vi "Overwrite Item.vi"(8 "error in (no error)":errorcluster, 9 "BetterTreeItem in":refnum<class "BetterItem.lvclass">, 10 "TreeItem Index":i32, 11 "BetterTreeHandle in":refnum<class "BetterTreeHandle.lvclass">) -> (0 "error out":errorcluster, 3 "BetterTreeHandle out":refnum<class "BetterTreeHandle.lvclass">)   [LabVIEW 2020, in "BetterDragAndDrop.lvlib" / "BetterTreeHandle.lvclass"]
uses:
  BetterTreeHandle.lvclass
  C:/DSCE code/Open-source/betterdraganddrop_GIT/Source/Classes/BetterHandle/BetterHandle.lvclass
  BetterTreeItem/BetterItem.lvclass
  BetterHandle/BetterHandle.lvclass/BetterHandle.ctl
  BetterTreeHandle.lvclass/BetterTreeHandle.ctl
  BetterTreeItem/BetterItem.lvclass/BetterItem.ctl
  BetterHandle/BetterHandle.lvclass
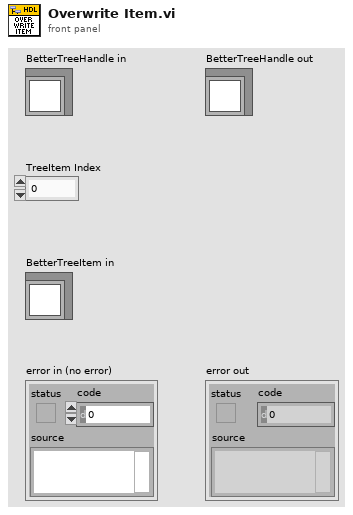
[diagram p1: front panel]
types:
  T1 = typedef "BetterDragAndDrop.lvlib/BetterTreeHandle.lvclass/TreeItem.ctl" = cluster{"Left Cell String":string, "Child Text":string[], "Child Tag":string, "Item Indent":i32, "Child Only?":bool, "Glyph Index":i32, "Font Color":u32}
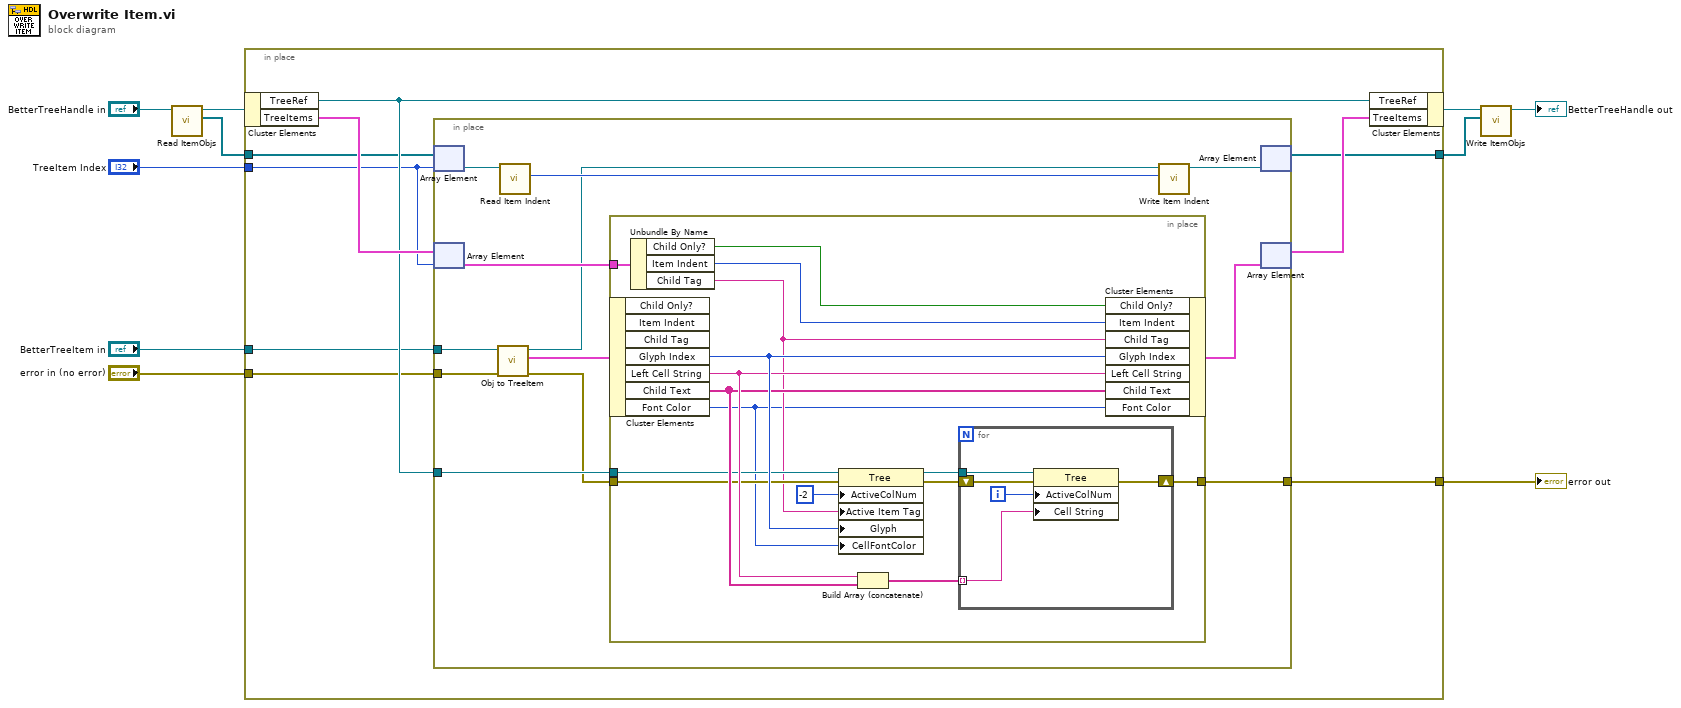
[diagram p0: block diagram]
diagram:
  n1 = call "Read ItemObjs.vi"("BetterHandle in"="BetterTreeHandle in") -> ("ItemObjs"=w4:refnum<class "BetterItem.lvclass">[], "BetterHandle out"=w5:refnum<class "BetterTreeHandle.lvclass">)  [unwired: 9 in]
  n2 = in-place {
    in-place-border: "error in (no error)" -> [w16]
    in-place-border: [w15] -> w8
    in-place-border: "TreeItem Index" -> [w14]
    in-place-border: "BetterTreeItem in" -> [w13]
    in-place-border: w4 -> [w12]
    in-place-border: [w11] -> w1
    n3 = in-place-cluster #1(w5) -> ("TreeRef"=w17:refnum<vi>, "TreeItems"=w19:T1[])
    n4 = in-place {
      in-place-border: w17 -> [w31]
      in-place-border: w13 -> [w24]
      in-place-border: w16 -> [w21]
      in-place-border: [w30] -> w15
      n5 = in-place-array #2(w12, w14) -> (w27:refnum<class "BetterItem.lvclass">)
      n6 = in-place-array #3(w19, w14) -> (w29:T1)
      n7 = call "Obj to TreeItem.vi"("error in (no error)"=w21, "BetterTreeItem in"=w24) -> ("error out"=w20:errorcluster, "Tree Control Item"=w22:T1, "BetterTreeItem out"=w23:refnum<class "BetterItem.lvclass">)  [unwired: 7 in]
      n8 = call "Read Item Indent.vi"("BetterTreeItem in"=w27) -> ("Item Indent"=w25:i32)  [unwired: 9 in, 1 out]
      n9 = in-place {
        in-place-border: w31 -> [w36]
        in-place-border: w20 -> [w35]
        in-place-border: [w43] -> w30
        in-place-border: w29 -> [w42]
        n10 = in-place-cluster #4(w22) -> ("Glyph Index"=w41:i32, "Left Cell String"=w40:string, "Child Text"=w39:string[], "Font Color"=w32:u32)  [unwired: 3 out]
        n11 = Unbundle By Name(w42) -> ("Child Only?"=w38:bool, "Item Indent"=w37:i32, "Child Tag"=w34:string)
        n12 = property class="Tree"(reference=w36, error in=w35, "ActiveColNum"=-2 ("Active Cell:Active Column Number"), "Active Item Tag"=w34, "Glyph"=w41, "CellFontColor"=w32) -> (reference out=w46:refnum<vi>, error out=w44:errorcluster)
        n13 = Build Array (concatenate)(w40, w39) -> (w45:string[])
        n14 = for {
          tunnel: w46 -> [w51]
          tunnel: w45 -> [w49] mode=indexing
          shift-right: [w47] -> w43
          shift-left: w44 -> [w48]
          i -> [w50]
          n15 = property class="Tree"(reference=w51, error in=w48, "ActiveColNum"=w50, "Cell String"=w49) -> (error out=w47:errorcluster)  [unwired: 1 out]
        }
        n16 = in-place-cluster #4("Child Only?"=w38, "Item Indent"=w37, "Child Tag"=w34, "Glyph Index"=w41, "Left Cell String"=w40, "Child Text"=w39, "Font Color"=w32) -> (w28:T1)
      }
      n17 = call "Write Item Indent.vi"("Item Indent"=w25, "BetterTreeItem in"=w23) -> ("BetterTreeItem out"=w26:refnum<class "BetterItem.lvclass">)  [unwired: 9 in]
      n18 = in-place-array #2(w26) -> (w11:refnum<class "BetterItem.lvclass">[])  [unwired: 1 out]
      n19 = in-place-array #3(w28) -> (w18:T1[])  [unwired: 1 out]
    }
    n20 = in-place-cluster #1("TreeRef"=w17, "TreeItems"=w18) -> (w3:refnum<class "BetterTreeHandle.lvclass">)
  }
  "error out" <- w8
  n21 = call "Write ItemObjs.vi"("ItemObjs"=w1, "BetterHandle in"=w3) -> ("BetterHandle out"=→"BetterTreeHandle out":refnum<class "BetterTreeHandle.lvclass">)  [unwired: 9 in]
